vi "SP Clear Calibration From INI File.vi"(8 "error in (no error)":errorcluster, 11 "Parameters to Measure":T1[](array[typedef]) {"Channel" min=1 max=99 step=1; "Parameter"."Stimulus Port" min=1 step=1; "Parameter"."Response Port" min=1 step=1}) -> (0 "error out":errorcluster)   [LabVIEW 2011]
uses:
  TypeDefs/SP Parameter to Measure.ctl
  TypeDefs/SP Parameter.ctl
  TypeDefs/SP Calibration State.ctl
  TypeDefs/SP Measurement Format.ctl
  <vilib>/Utility/config.llb/NI_LVConfig.lvlib
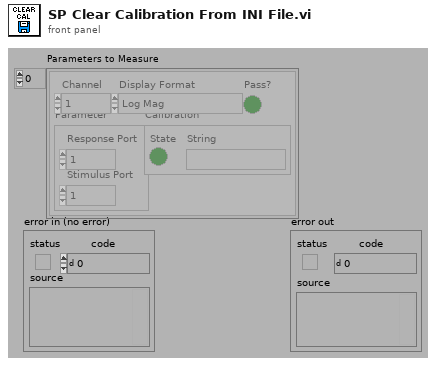
[diagram p1: front panel]
types:
  T1 = typedef "SP Parameter to Measure.ctl" = cluster{"Channel":i8, "Parameter":T2, "Calibration":T3, "Display Format":T4, "Pass?":bool}
  T2 = typedef "SP Parameter.ctl" = cluster{"Stimulus Port":i8, "Response Port":i8}
  T3 = typedef "SP Calibration State.ctl" = cluster{"State":bool, "String":string}
  T4 = typedef "SP Measurement Format.ctl" = enum32{"Log Mag", "Phase", "Delay", "Smith (R+jX)", "Polar (Re/Im)", "Linear Mag", "SWR", "Real", "Imaginary", "Smith (Lin/Phase)", "Smith (Log/Phase)", "Smith (Real/Imag)", "Smith (G+jB)", "Polar (Lin/Phase)", "Polar (Log/Phase)", "Expanded Phase", "Positive Phase", "Inverted Smith", "Unwrapped Phase", "Power Out", "Power In", "Linear Mag/Phase", "Log Mag/Phase", "Real/Imaginary"}
  T5 = typedef "NI_LVConfig.lvlib/Config Data RefNum.ctl" = refnum<k1>
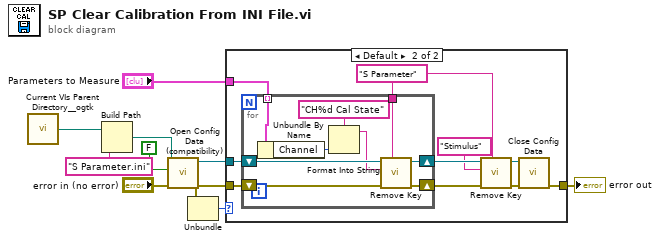
[diagram p0: block diagram]
diagram:
  n1 = call "Current VIs Parent Directory__ogtk.vi"() -> ("Parent Directory (+ Relative)"=w1:path)  [unwired: 5 in]
  n2 = Build Path(base path=w1, name or relative path="S Parameter.ini") -> (appended path=w3:path)
  n3 = call <vilib>:"Open Config Data (compatibility).vi"("error in (no error)"="error in (no error)", "create file if necessary (T)"=FALSE ("create file if necessary? (T)"), "configuration file path"=w3) -> ("error out"=w6:errorcluster, "refnum"=w10:T5)  [unwired: 6 in, 1 out]
  n4 = Unbundle(w6) -> ("code"=w5:i32)  [unwired: 2 out]
  n5 = case shown="Default" w5 {
    tunnel: w6 -> [_ w20]
    tunnel: w10 -> [_ w15]
    tunnel: [_ w14] -> w8
    tunnel: "Parameters to Measure" -> [_ w11]
    frame 7 {
    }
    frame Default {
      w12 = "S Parameter" ("name or relative path")
      n6 = for {
        shift-right: [w27] -> w16
        shift-left: w15 -> [w26]
        shift-right: [w28] -> w19
        shift-left: w20 -> [w29]
        tunnel: w12 -> [w25]
        tunnel: w11 -> [w24] mode=indexing
        n7 = Unbundle By Name(w24) -> ("Channel"=w23:i8)
        n8 = Format Into String(format string="CH%d Cal State" ("name or relative path"), w23) -> (resulting string=w22:string)  [unwired: 2 in, 1 out]
        n9 = call <vilib>:"Remove Key.vi"("section"=w25, "error in (no error)"=w29, "key"=w22, "refnum"=w26) -> ("error out"=w28:errorcluster, "refnum out"=w27:T5)  [unwired: 6 out]
      }
      n10 = call <vilib>:"Remove Key.vi"("section"=w12, "error in (no error)"=w19, "key"="Stimulus" ("name or relative path"), "refnum"=w16) -> ("error out"=w18:errorcluster, "refnum out"=w17:T5)  [unwired: 6 out]
      n11 = call <vilib>:"Close Config Data.vi"("error in (no error)"=w18, "refnum"=w17) -> ("error out"=w14:errorcluster)  [unwired: 1 in, 8 out]
    }
  }
  "error out" <- w8
